vi "Lab19_FolderQueue.vi"() -> ()   [LabVIEW 2022 SP3]
panel:
  out "File in both A and B":variant[](array[variant])
  out "File in A not B":variant[](array[variant])
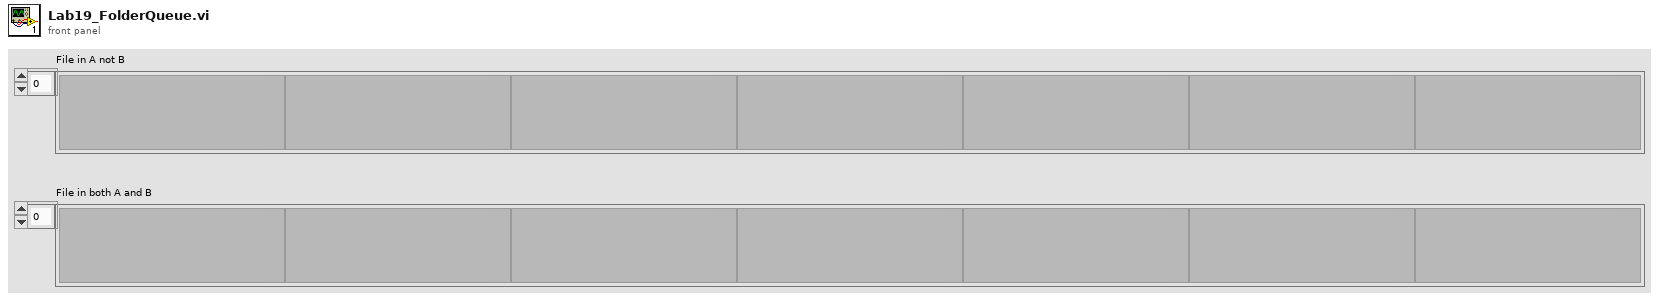
[diagram p1: front panel]
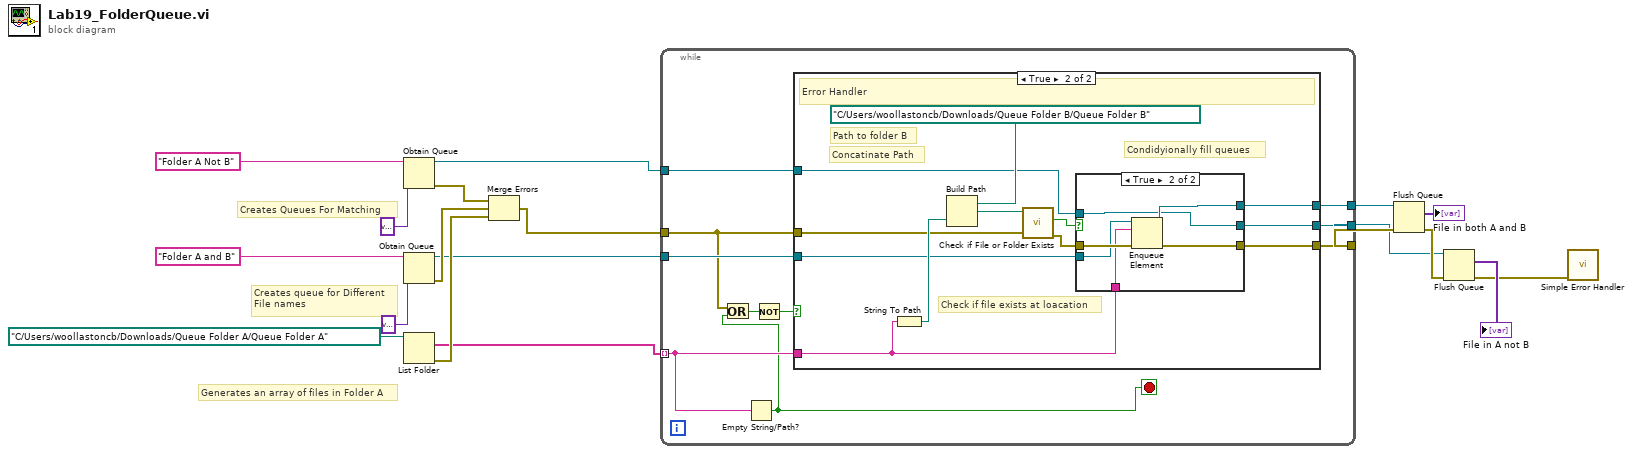
[diagram p0: block diagram]
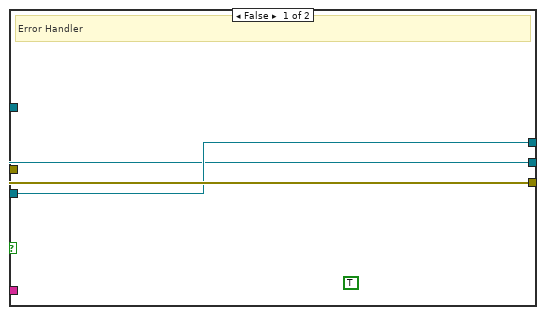
[diagram p2: hidden frame]
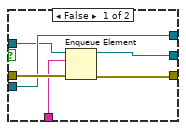
[diagram p3: hidden frame]
diagram:
  # "Generates an array of files in Folder A"
  # "Creates queue for Different\nFile names"
  # "Creates Queues For Matching"
  n1 = Obtain Queue(name (unnamed)="Folder A Not B", element data type=variant) -> (queue out=w10:refnum<queue>, error out=w16:errorcluster)  [unwired: 3 in, 1 out]
  n2 = Obtain Queue(name (unnamed)="Folder A and B", element data type=variant) -> (queue out=w11:refnum<queue>, error out=w15:errorcluster)  [unwired: 3 in, 1 out]
  n3 = List Folder(path=path "C:/Users/woollastoncb/Downloads/Queue Folder A/Queue Folder A") -> (filenames=w12:string[], error out=w14:errorcluster)  [unwired: 3 in, 2 out]
  n4 = Merge Errors(w16, w15, w14) -> (w13:errorcluster)
  n5 = while {
    tunnel: w12 -> [w29] mode=indexing
    tunnel: w13 -> [w21]
    tunnel: w11 -> [w28]
    tunnel: w10 -> [w27]
    tunnel: [w26] -> w7
    tunnel: [w25] -> w4
    tunnel: [w24] -> w6
    stop <- w22 stop-if-true
    n6 = Empty String/Path?(string/path=w29) -> (empty?=w22:bool)
    n7 = Or(x=w21, y=w22) -> (x .or. y?=w23:bool)
    n8 = Not(x=w23) -> (.not. x?=w20:bool)
    n9 = case shown="True" w20 {
      tunnel: w29 -> [_ w33]
      tunnel: w21 -> [w32 w40]
      tunnel: w28 -> [w31 w38]
      tunnel: w27 -> [w30 w37]
      tunnel: [w31 w36] -> w26
      tunnel: [w30 w35] -> w25
      tunnel: [w32 w34] -> w24
      frame False {
        (unwired) TRUE
        # "Error Handler"
      }
      frame True {
        # "Condidyionally fill queues"
        # "Check if file exists at loacation"
        # "Concatinate Path"
        # "Path to folder B"
        # "Error Handler"
        n10 = String To Path(string=w33) -> (path=w44:path)
        n11 = Build Path(base path=path "C:/Users/woollastoncb/Downloads/Queue Folder B/Queue Folder B", name or relative path=w44) -> (appended path=w42:path)
        n12 = call <vilib>:"Check if File or Folder Exists.vi"("error in (no error)"=w40, "path"=w42) -> ("error out"=w39:errorcluster, "file or folder exists?"=w41:bool)  [unwired: 7 in, 1 out]
        n13 = case shown="True" w41 {
          tunnel: w39 -> [w50 w56]
          tunnel: [w49 w55] -> w34
          tunnel: w38 -> [w48 w54]
          tunnel: [w48 w53] -> w36
          tunnel: w37 -> [w47 w52]
          tunnel: [w46 w52] -> w35
          tunnel: w33 -> [w45 w51]
          frame False {
            n14 = Enqueue Element(queue=w47, element=w45, error in (no error)=w50) -> (queue out=w46:refnum<queue>, error out=w49:errorcluster)  [unwired: 1 in, 1 out]
          }
          frame True {
            n15 = Enqueue Element(queue=w54, element=w51, error in (no error)=w56) -> (queue out=w53:refnum<queue>, error out=w55:errorcluster)  [unwired: 1 in, 1 out]
          }
        }
      }
    }
  }
  n16 = Flush Queue(queue=w7, error in (no error)=w6) -> (remaining elements=→"File in both A and B":variant[], error out=w5:errorcluster)  [unwired: 1 out]
  n17 = Flush Queue(queue=w4, error in (no error)=w5) -> (remaining elements=→"File in A not B":variant[], error out=w2:errorcluster)  [unwired: 1 out]
  n18 = call <vilib>:"Simple Error Handler.vi"("error in (no error)"=w2) -> ()  [unwired: 4 in, 5 out]
